vi "ROE200_GetCurrentPosition.vi"(8 "error in (no error)":errorcluster, 11 "VISA resource name":refnum<visa-resource-name>) -> (0 "Z Position":u32, 1 "Y Position":u32, 2 "X Position":u32, 3 "Active Drive":u8, 4 "error out":errorcluster, 5 "VISA resource  out":refnum<visa-resource-name>, 6 "error in GetCurrentPosition":bool)   [LabVIEW 2019]
panel:
  out "read buffer":string
  out "return count each":u32
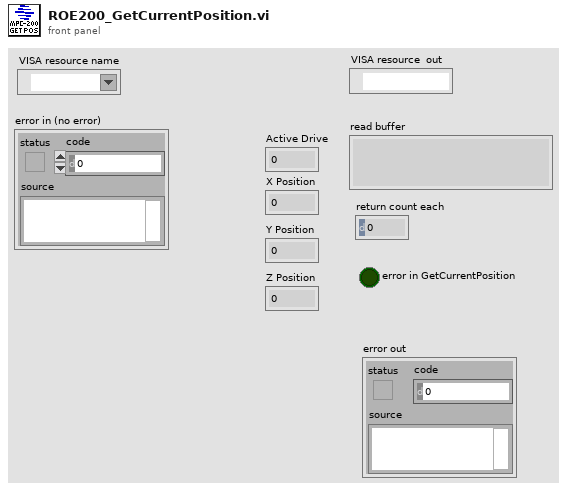
[diagram p1: front panel]
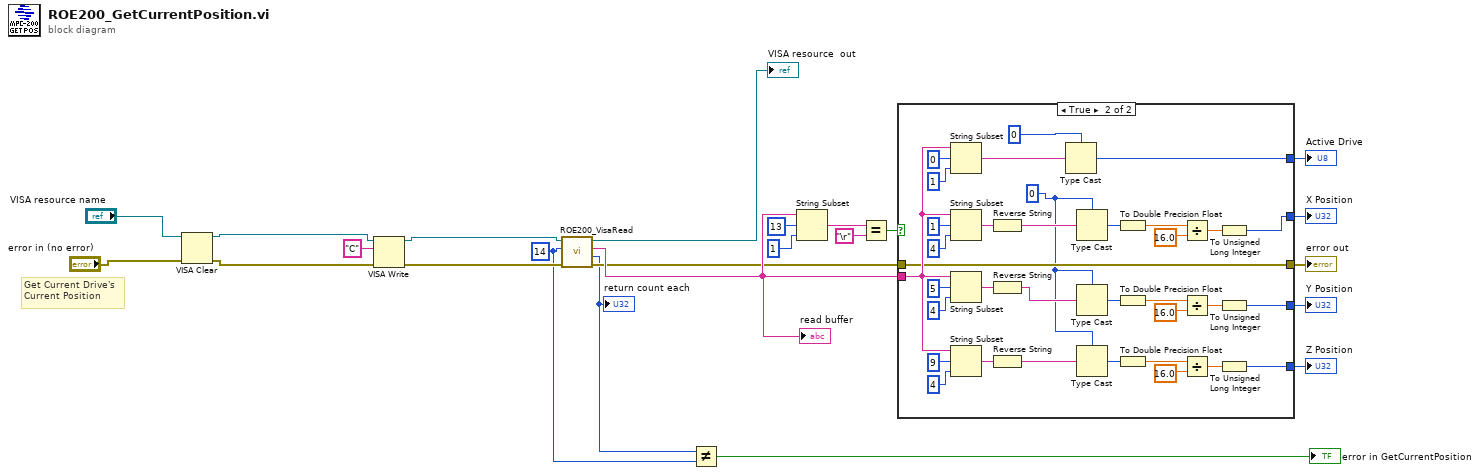
[diagram p0: block diagram]
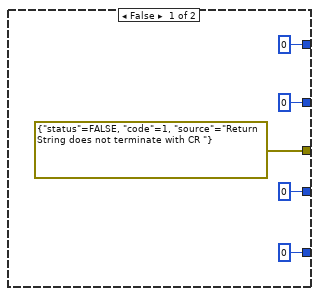
[diagram p2: hidden frame]
diagram:
  w2 = u32 14 ("Expected Bytes")
  # "Get Current Drive's\nCurrent Position"
  n1 = VISA Clear(VISA resource name="VISA resource name", error in (no error)="error in (no error)") -> (VISA resource name out=w4:refnum<visa-resource-name>, error out=w6:errorcluster)
  n2 = VISA Write(VISA resource name=w4, write buffer="C", error in (no error)=w6) -> (VISA resource name out=w21:refnum<visa-resource-name>, error out=w22:errorcluster)  [unwired: 1 out]
  n3 = call "ROE200_VisaRead.vi"("error in (no error)"=w22, "Expected Bytes"=w2, "Visa Reference In"=w21) -> ("error out"=w10:errorcluster, "return count"=w3:u32, "read buffer"=w14:string, "VISA resource  out"=→"VISA resource  out":refnum<visa-resource-name>)  [unwired: 5 in]
  "return count each" <- w3
  "read buffer" <- w14
  n4 = Not Equal?(x=w3, y=w2) -> (x != y?=→"error in GetCurrentPosition":bool)
  n5 = String Subset(string=w14, offset (0)=13, length (rest)=1 ("length (rest)")) -> (substring=w17:string)
  n6 = Equal?(x=w17, y="\r") -> (x = y?=w15:bool)
  n7 = case shown="True" w15 {
    tunnel: w14 -> [_ w36]
    tunnel: [u32 0 w35] -> w13
    tunnel: [u32 0 w34] -> w12
    tunnel: [u32 0 w33] -> w11
    tunnel: w10 -> [_ w32]
    tunnel: [errorcluster {"status"=FALSE, "code"=1, "source"="Return String does not terminate with CR "} ("error out") w32] -> w9
    tunnel: [i8 0 w31] -> w8
    frame False {
    }
    frame True {
      w29 = u32 0
      n8 = String Subset(string=w36, offset (0)=0, length (rest)=1 ("length (rest)")) -> (substring=w61:string)
      n9 = String Subset(string=w36, offset (0)=1, length (rest)=4 ("length (rest)")) -> (substring=w58:string)
      n10 = String Subset(string=w36, offset (0)=5, length (rest)=4 ("length (rest)")) -> (substring=w55:string)
      n11 = String Subset(string=w36, offset (0)=9, length (rest)=4 ("length (rest)")) -> (substring=w49:string)
      n12 = Reverse String(1:w58) -> (0:w51:string)
      n13 = Reverse String(1:w55) -> (0:w50:string)
      n14 = Reverse String(1:w49) -> (0:w37:string)
      n15 = Type Cast(type=u8 0, x=w61) -> (*(type *) &x=w31:u8)
      n16 = Type Cast(type=w29, x=w51) -> (*(type *) &x=w52:u32)
      n17 = Type Cast(type=w29, x=w50) -> (*(type *) &x=w39:u32)
      n18 = Type Cast(type=w29, x=w37) -> (*(type *) &x=w38:u32)
      n19 = To Double Precision Float(number=w52) -> (double precision float=w47:dbl)
      n20 = To Double Precision Float(number=w39) -> (double precision float=w44:dbl)
      n21 = To Double Precision Float(number=w38) -> (double precision float=w41:dbl)
      n22 = Divide(x=w47, y=16.0) -> (x/y=w48:dbl)
      n23 = Divide(x=w44, y=16.0) -> (x/y=w45:dbl)
      n24 = Divide(x=w41, y=16.0) -> (x/y=w42:dbl)
      n25 = To Unsigned Long Integer(number=w48) -> (unsigned 32bit integer=w35:u32)
      n26 = To Unsigned Long Integer(number=w45) -> (unsigned 32bit integer=w34:u32)
      n27 = To Unsigned Long Integer(number=w42) -> (unsigned 32bit integer=w33:u32)
    }
  }
  "error out" <- w9
  "X Position" <- w13
  "Y Position" <- w12
  "Z Position" <- w11
  "Active Drive" <- w8
